vi "PowerOff.vi"(0 "Universal Robot.lvclass in":refnum<class "Universal Robot.lvclass">, 5 "error in (no error)":errorcluster) -> (14 "Universal Robot.lvclass out":refnum<class "Universal Robot.lvclass">, 19 "error out":errorcluster)   [LabVIEW 2019, in "Universal Robot.lvclass"]
uses:
  Universal Robot.lvclass
  Universal Robot.lvclass/Universal Robot.ctl
  RobotMode.ctl
  Client Interfaces/Dashboard Server/Dashboard Server.lvclass
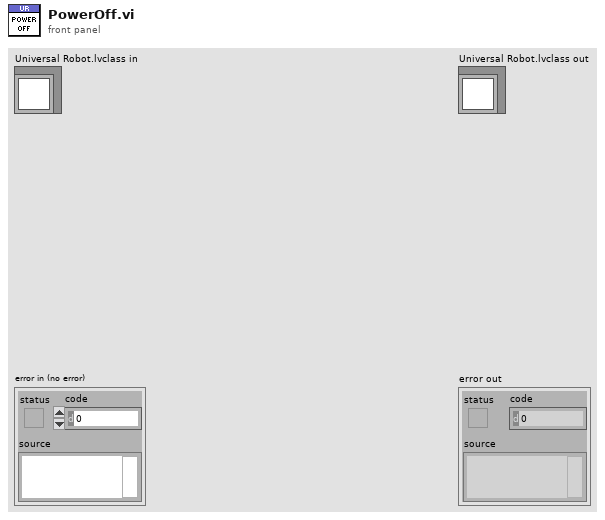
[diagram p1: front panel]
types:
  T1 = typedef "Universal Robot.lvclass/RobotMode.ctl" = enum16{"INVALID", "NO_CONTROLLER", "DISCONNECTED", "CONFIRM_SAFETY", "BOOTING", "POWER_OFF", "POWER_ON", "IDLE", "BACKDRIVE", "RUNNING"}
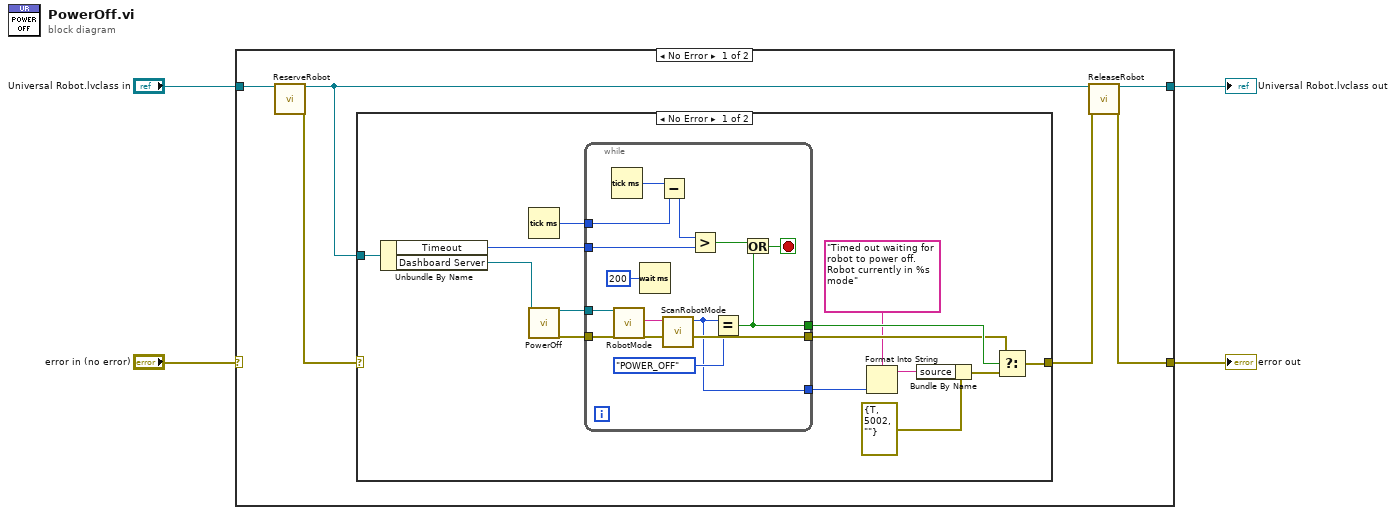
[diagram p0: block diagram]
diagram:
  n1 = case shown="No Error" "error in (no error)" {
    selector: "error in (no error)" -> [_ w41]
    tunnel: [w5 w41] -> w3
    tunnel: "Universal Robot.lvclass in" -> [w9 w40]
    tunnel: [w10 w40] -> w1
    frame No Error {
      n2 = call "ReserveRobot.vi"("Universal Robot.lvclass in"=w9) -> ("Universal Robot.lvclass out"=w8:refnum<class "Universal Robot.lvclass">, "error out"=w7:errorcluster)  [unwired: 17 in]
      n3 = case shown="No Error" w7 {
        selector: w7 -> [_ w39]
        tunnel: w8 -> [w12 _]
        tunnel: [w11 w39] -> w6
        frame No Error {
          n4 = Unbundle By Name(w12) -> ("Timeout"=w24:u32, "Dashboard Server"=w13:refnum<class "Dashboard Server.lvclass">)
          n5 = Tick Count (ms)() -> (millisecond timer value=w23:u32)
          n6 = call-dynamic "PowerOff.vi"("DashboardServer in"=w13) -> ("DashboardServer out"=w14:refnum<class "Dashboard Server.lvclass">, "error out"=w15:errorcluster)  [unwired: 17 in]
          n7 = while {
            tunnel: w14 -> [w37]
            tunnel: w15 -> [w38]
            tunnel: [w36] -> w21
            tunnel: w24 -> [w34]
            tunnel: w23 -> [w33]
            tunnel: [w28] -> w22
            tunnel: [w25] -> w20
            stop <- w29 stop-if-true
            n8 = Tick Count (ms)() -> (millisecond timer value=w32:u32)
            n9 = call-dynamic "RobotMode.vi"("DashboardServer in"=w37, "error in (no error)"=w38) -> ("robotMode"=w27:string, "error out"=w36:errorcluster)  [unwired: 15 in, 1 out]
            n10 = Wait (ms)(milliseconds to wait=u32 200) -> ()  [unwired: 1 out]
            n11 = Subtract(x=w32, y=w33) -> (x-y=w31:u32)
            n12 = call "ScanRobotMode.vi"("robotMode in"=w27) -> ("robotMode out"=w25:T1)  [unwired: 10 in]
            n13 = Greater?(x=w31, y=w34) -> (0:w30:bool)
            n14 = Equal?(x=w25, y=RobotMode."POWER_OFF") -> (x = y?=w28:bool)
            n15 = Or(x=w30, y=w28) -> (x .or. y?=w29:bool)
          }
          n16 = Format Into String(format string="Timed out waiting for robot to power off. Robot currently in %s mode", w20) -> (resulting string=w18:string)  [unwired: 2 in, 1 out]
          n17 = Bundle By Name(cluster=errorcluster {"status"=TRUE, "code"=5002, "source"=""} ("error constant"), "source"=w18) -> (w17:errorcluster)
          n18 = Select(t=w21, s=w22, f=w17) -> (s? t:f=w11:errorcluster)
        }
        frame Error {
        }
      }
      n19 = call "ReleaseRobot.vi"("Universal Robot.lvclass in"=w8, "error in (no error)"=w6) -> ("Universal Robot.lvclass out"=w10:refnum<class "Universal Robot.lvclass">, "error out"=w5:errorcluster)  [unwired: 16 in]
    }
    frame Error {
    }
  }
  "error out" <- w3
  "Universal Robot.lvclass out" <- w1
